vi "(auto) Skip same balls(SubVI).vi"(10 "Circles Calibrated (Shape Detection 1)":T1(array[cluster]), 11 "balls counter":i32) -> (2 "balls coutnter Out":i32, 3 "arrOut":i32[](array[numeric]))   [LabVIEW 2017]
uses:
  <vilib>/imath/engines/lvmath2/RunTimeEngine/NodeEndStatement/NIMS_NodeEndStatement_Output.vi
  <instcachedir>/0/NIMS_NodeEndStatement_Output_53EC0D466D134D7ABD903AC30B43404B.lvgen/NIMS_NodeEndStatement_Output_53EC0D466D134D7ABD903AC30B43404B_012.vi
  <instcachedir>/0/NIMS_NodeEndStatement_Output_53EC0D466D134D7ABD903AC30B43404B.lvgen/NIMS_NodeEndStatement_Output_53EC0D466D134D7ABD903AC30B43404B_010.vi
  <vilib>/imath/engines/lvmath2/RunTimeEngine/ErrorHandling/NIMS_Finalize Error.vi
panel:
  in  "range":dbl
  out "y1":sgl
  out "x1":sgl
  out "y2":sgl
  out "x2":sgl
  out "indx":i32
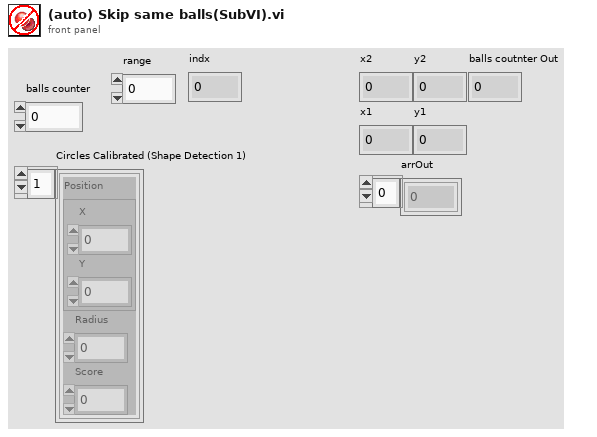
[diagram p1: front panel]
types:
  T1 = cluster{"Position":cluster{"X":sgl, "Y":sgl}, "Radius":dbl, "Score":dbl}[]
  T2 = cluster{"Position":cluster{"X":sgl, "Y":sgl}, "Radius":dbl, "Score":dbl}
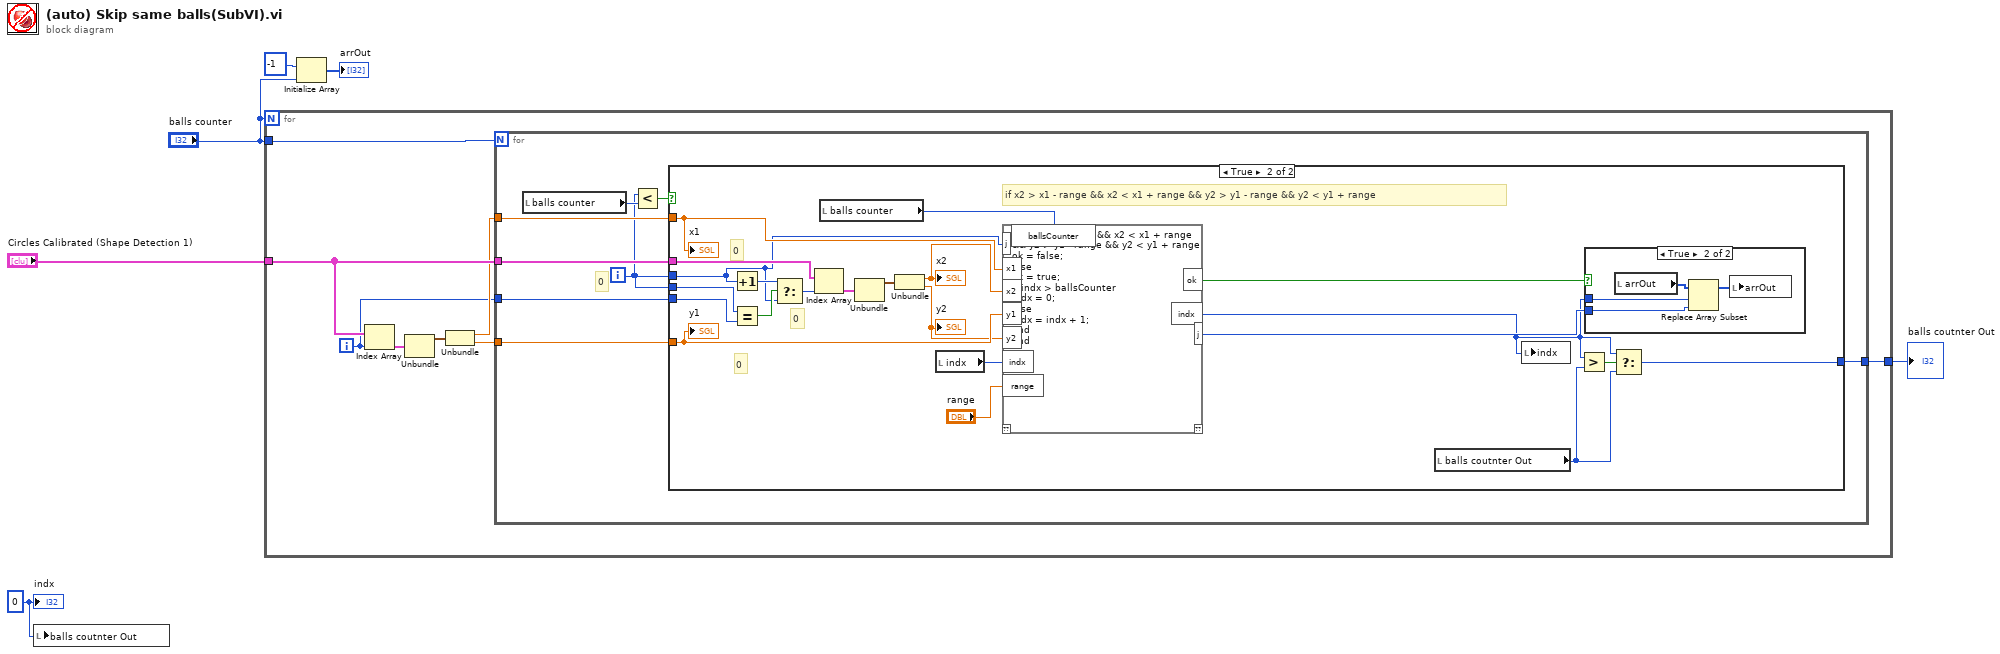
[diagram p0: block diagram]
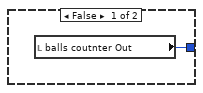
[diagram p2: hidden frame]
diagram:
  w1 = 0 ("indx")
  n1 = local write "balls coutnter Out"(w1) -> ()
  n2 = for {
    N: "balls counter" -> [_]
    tunnel: "Circles Calibrated (Shape Detection 1)" -> [w12]
    tunnel: "balls counter" -> [w8]
    tunnel: [w9] -> w2
    i -> [w7]
    n3 = Index Array(array=w12, index=w7) -> (element=w14:T2)
    n4 = Unbundle(w14) -> ("Position"=w13:cluster{"X":sgl, "Y":sgl})  [unwired: 2 out]
    n5 = Unbundle(w13) -> ("X"=w11:sgl, "Y"=w10:sgl)
    n6 = for {
      N: w8 -> [_]
      tunnel: w12 -> [w22]
      tunnel: w11 -> [w21]
      tunnel: w10 -> [w20]
      tunnel: [w19] -> w9
      tunnel: w7 -> [w16]
      i -> [w15]
      # "0"
      n7 = local read "balls counter"() -> (w18:i32)
      n8 = Less?(x=w15, y=w18) -> (x < y?=w17:bool)
      n9 = case shown="True" w17 {
        tunnel: w22 -> [_ w45]
        tunnel: w21 -> [_ w42]
        tunnel: w20 -> [_ w41]
        tunnel: w16 -> [_ w35]
        tunnel: w15 -> [_ w32]
        tunnel: w15 -> [_ w30]
        tunnel: [w23 w28] -> w19
        frame False {
          n10 = local read "balls coutnter Out"() -> (w23:i32)
        }
        frame True {
          # "0"
          # "0"
          # "0"
          # "if x2 > x1 - range && x2 < x1 + range && y2 > y1 - range && y2 < y1 + range"
          n11 = Increment(x=w30) -> (x+1=w33:i32)
          n12 = Equal?(x=w32, y=w35) -> (x = y?=w34:bool)
          n13 = Select(t=w33, s=w34, f=w30) -> (s? t:f=w31:i32)
          n14 = Index Array(array=w45, index=w31) -> (element=w44:T2)
          n15 = local read "balls counter"() -> (w24:i32)
          n16 = Unbundle(w44) -> ("Position"=w43:cluster{"X":sgl, "Y":sgl})  [unwired: 2 out]
          n17 = Unbundle(w43) -> ("X"=w40:sgl, "Y"=w39:sgl)
          "x2" <- w40
          "y2" <- w39
          n18 = local read "indx"() -> (w29:i32)
          n19 = mathscript code="if x2 > x1 - range && x2 < x1 + range && y2 > y1 - range && y2 < y1 + range\nok = false;\nelse\nok = true;\nif indx > ballsCounter\nindx = 0;\nelse\nindx = indx + 1;\nend\nend"("x1"=w42, "x2"=w40, "y1"=w41, "y2"=w39, "indx"=w29, "range"="range", "j"=w30, "ballsCounter"=w24) -> ("ok"=w37:bool, "indx"=w25:i32, "j"=w36:i32)  [unwired: 1 in, 1 out]
          n20 = local read "balls coutnter Out"() -> (w26:i32)
          n21 = local write "indx"(w25) -> ()
          n22 = Greater?(x=w25, y=w26) -> (0:w27:bool)
          n23 = case shown="True" w37 {
            tunnel: w25 -> [_ w47]
            tunnel: w36 -> [_ w46]
            frame False {
            }
            frame True {
              n24 = local read "arrOut"() -> (w48:i32[])
              n25 = Replace Array Subset(array=w48, new element=w46, index=w47) -> (w49:i32[])
              n26 = local write "arrOut"(w49) -> ()
            }
          }
          n27 = Select(t=w25, s=w27, f=w26) -> (s? t:f=w28:i32)
          "x1" <- w42
          "y1" <- w41
        }
      }
    }
  }
  "balls coutnter Out" <- w2
  n28 = Initialize Array(-1 ("element"), "balls counter") -> (→"arrOut":i32[])
  "indx" <- w1
